vi "CSM - List Modules.vi"(8 "Error in":errorcluster caption="Error in (no error)", 9 "All?":bool) -> (0 "Error out":errorcluster, 3 "Module Names":string[](array[string]))   [LabVIEW 2020, in "Communicable State Machine.lvlib"]
doc: "List all CSM Modules alive in system.\n\n<b>Inputs:</b>\n - <b>Exclude Standalone CSM(T)</b>: 'TRUE' to exclude standalone CSM module, and 'FALSE' to include them.\n - <b>Error in</b>: Error cluster\n\n<b>Outputs:</b>\n - <b>Module Names</b>: Module Names\n - <b>Error out</b>: Error cluster"
uses:
  Communicable State Machine.lvlib
  _CSMOFGVOPER.ctl
  global-CSMQ FGV Change Flag.vi
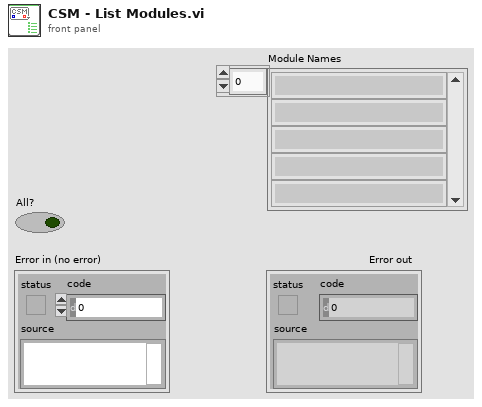
[diagram p1: front panel]
types:
  T1 = typedef "Communicable State Machine.lvlib/_CSMOFGVOPER.ctl" = enum16{"Create If not Exist", "Get By Name", "List", "Check If Name Exists", "Release", "Module Status", "Create Status Event Handler", "Destroy Status Event Handler"}
  T2 = typedef "Communicable State Machine.lvlib/_CSMObj.ctl" = cluster{"Requested Name":string, "Module Name":string, "Mode":T3, "Queue":refnum<class "Priority Queue.lvclass">, "CSM-Data":refnum<data-value>, "User Event":refnum<user-event>, "Status Change Event":refnum<user-event>, "Allowed Messages":string[], "Mode-Data":refnum<data-value>, "Group Name":string, "Exit Event":refnum<user-event>}
  T3 = typedef "Communicable State Machine.lvlib/_CSM_MODE.ctl" = enum16{"Not Exist", "Stand Alone", "CSM", "Worker Agent", "Worker", "Chain", "Chain Node"}
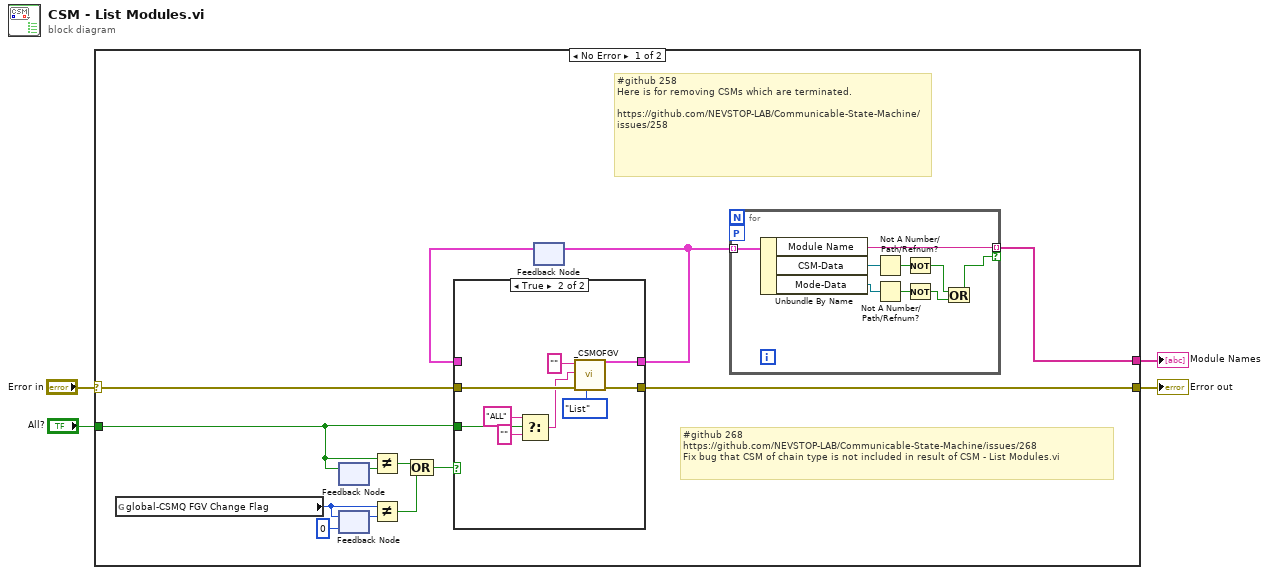
[diagram p0: block diagram]
diagram:
  n1 = case shown="No Error" "Error in" {
    selector: "Error in" -> [w17 w38]
    tunnel: [w16 w38] -> w3
    tunnel: "All?" -> [w12 _]
    tunnel: [w5 _] -> w1
    frame No Error {
      # "#github 268\nhttps://github.com/NEVSTOP-LAB/Communicable-State-Machine/issues/268\nFix bug that CSM of chain type is not included in result of CSM - List Modules.vi"
      # "#github 258\nHere is for removing CSMs which are terminated.\n\nhttps://github.com/NEVSTOP-LAB/Communicable-State-Machine/issues/258"
      n2 = global read "global-CSMQ FGV Change Flag.vi" "global-CSMQ FGV Change Flag"() -> (w14:u64)
      n3 = feedback #1() -> (w13:bool)  [unwired: 1 in]
      n4 = feedback-in #1(w12) -> ()
      n5 = feedback #2(u64 0 ("global-CSMQ FGV Change Flag")) -> (w15:u64)
      n6 = feedback-in #2(w14) -> ()
      n7 = Not Equal?(x=w12, y=w13) -> (x != y?=w11:bool)
      n8 = Not Equal?(x=w14, y=w15) -> (x != y?=w10:bool)
      n9 = Compound Arithmetic op=OR(w11, w10) -> (w9:bool)
      n10 = feedback #3() -> (w8:T2[])  [unwired: 1 in]
      n11 = case shown="True" w9 {
        tunnel: w17 -> [w28 w37]
        tunnel: [w28 w36] -> w16
        tunnel: w12 -> [_ w35]
        tunnel: [w27 w29] -> w6
        tunnel: w8 -> [w27 _]
        frame False {
        }
        frame True {
          n12 = Select(t="ALL" ("Name(\"\" to use uuid) in"), s=w35, f="" ("Name(\"\" to use uuid) in")) -> (s? t:f=w30:string)
          n13 = call "_CSMOFGV.vi"("Operation"=_CSMOFGVOPER."List", "Error in"=w37, "Reference"=w30, "Name(\"\" to use uuid) in"="" ("Name(\"\" to use uuid) in")) -> ("Error out"=w36:errorcluster, "Array"=w29:T2[])  [unwired: 5 in, 1 out]
        }
      }
      n14 = feedback-in #3(w6) -> ()
      n15 = for {
        tunnel: w6 -> [w26] mode=indexing
        tunnel: [w25] -> w5 mode=indexing if=w23
        workers-P: _ -> [_]
        n16 = Unbundle By Name(w26) -> ("Module Name"=w25:string, "CSM-Data"=w20:refnum<data-value>, "Mode-Data"=w19:refnum<data-value>)
        n17 = Not A Number/Path/Refnum?(number/path/refnum=w20) -> (NaN/Path/Refnum?=w24:bool)
        n18 = Not A Number/Path/Refnum?(number/path/refnum=w19) -> (NaN/Path/Refnum?=w21:bool)
        n19 = Not(x=w24) -> (.not. x?=w22:bool)
        n20 = Not(x=w21) -> (.not. x?=w18:bool)
        n21 = Or(x=w22, y=w18) -> (x .or. y?=w23:bool)
      }
    }
    frame Error {
    }
  }
  "Error out" <- w3
  "Module Names" <- w1
